vi "Execute_Command.vi"(11 "Command":string) -> (0 "error out":errorcluster, 2 "File to run":string, 3 "Input":string)   [LabVIEW 2012]
uses:
  <vilib>/Rock Robotics/WPI/DriverStation/DriverStationLCD/WPI_DriverStationLCDLCDLine.ctl
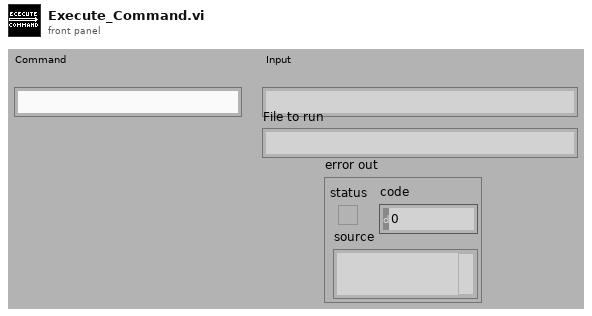
[diagram p1: front panel]
types:
  T1 = typedef "WPI_DriverStationLCDLCDLine.ctl" = enum16{"Main - Line 1", "User - Line 2", "User - Line 3", "User - Line 4", "User - Line 5", "User - Line 6"}
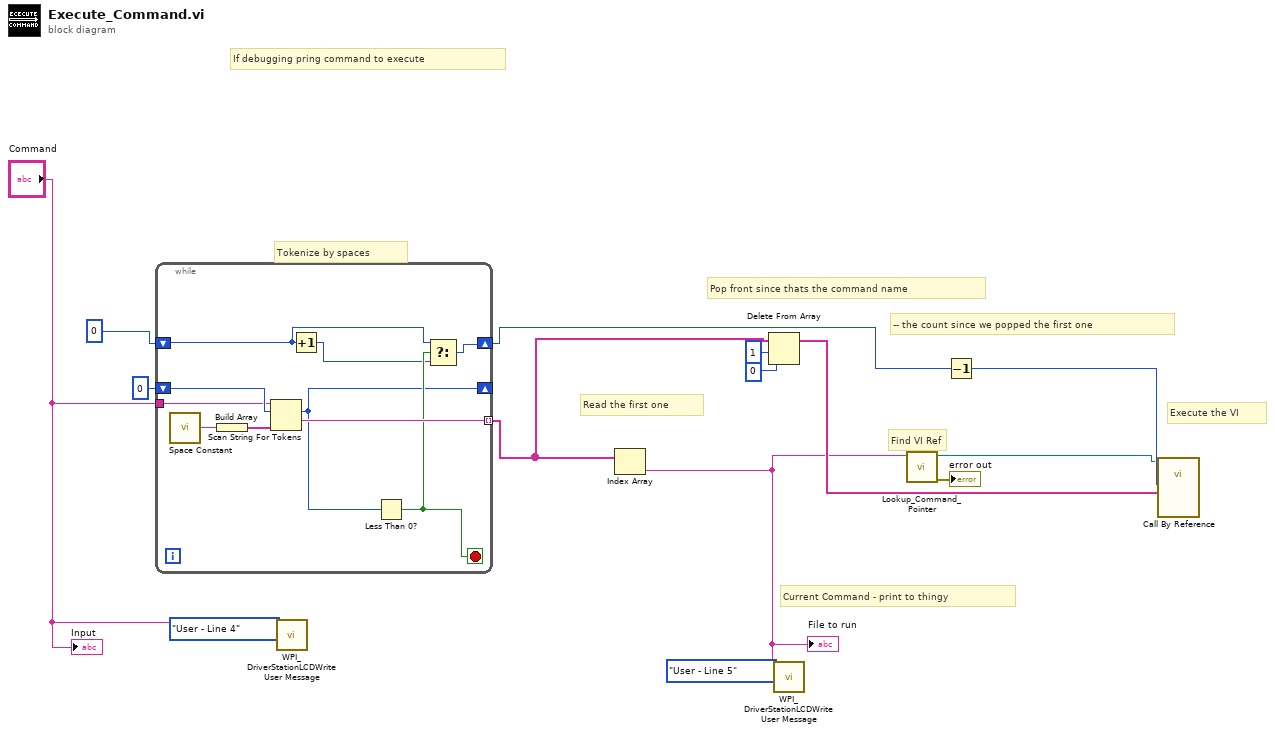
[diagram p0: block diagram]
diagram:
  # "Current Command - print to thingy"
  # "If debugging pring command to execute"
  # "Execute the VI"
  # "-- the count since we popped the first one"
  # "Pop front since thats the command name"
  # "Find VI Ref"
  # "Read the first one"
  # "Tokenize by spaces"
  n1 = while {
    shift-right: [w15] -> _
    shift-left: 0 ("offset past token") -> [w24]
    tunnel: "Command" -> [w23]
    tunnel: [w22] -> w8 mode=indexing
    shift-right: [w18] -> w11
    shift-left: u8 0 -> [w20]
    stop <- w21 stop-if-true
    n2 = call <vilib>:"Space Constant.vi"() -> ("String"=w17:string)
    n3 = Build Array(w17) -> (w16:string[])
    n4 = Scan String For Tokens(6:w16, 8:w24, 9:w23) -> (1:w22:string, 2:w15:i32)  [unwired: 5 out]
    n5 = Increment(x=w20) -> (x+1=w19:u8)
    n6 = Less Than 0?(x=w15) -> (x < 0?=w21:bool)
    n7 = Select(t=w20, s=w21, f=w19) -> (s? t:f=w18:u8)
  }
  n8 = call <vilib>:"WPI_DriverStationLCDWrite User Message.vi"("line text"="Command", "line"=WPI_DriverStationLCDLCDLine."User - Line 4") -> ()  [unwired: 3 in, 11 out]
  n9 = Index Array(array=w8) -> (element=w3:string)  [unwired: 1 in]
  "File to run" <- w3
  n10 = Delete From Array(array=w8, length=1, index=0) -> (array with subset deleted=w9:string[])  [unwired: 1 out]
  n11 = call <vilib>:"WPI_DriverStationLCDWrite User Message.vi"("line text"=w3, "line"=WPI_DriverStationLCDLCDLine."User - Line 5") -> ()  [unwired: 3 in, 11 out]
  n12 = call "Lookup_Command_Pointer.vi"("refnum name"=w3) -> ("error out"=→"error out":errorcluster, "VI Refnum Out"=w6:refnum<vi>)  [unwired: 9 in]
  n13 = Decrement(x=w11) -> (x-1=w10:u8)
  n14 = call-by-ref "?"(reference=w6, "argv"=w9, "args"=w10) -> ()  [unwired: 11 in, 2 out]
  "Input" <- "Command"
